vi "Plot Generator.vi"(7 "Frequency (Hz)":dbl, 8 "Count in":i32, 9 "Noise Level":dbl, 10 "Amplitude":dbl, 11 "DC":dbl) -> (2 "Numeric out":dbl)   [LabVIEW 2015]
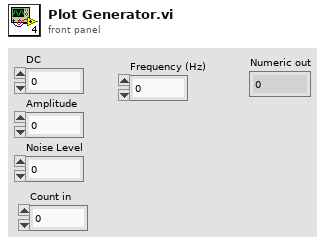
[diagram p1: front panel]
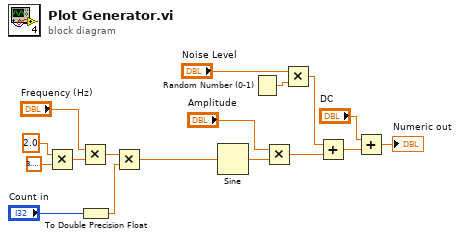
[diagram p0: block diagram]
diagram:
  n1 = Multiply(x=2.0, y=3.141592653589793) -> (x*y=w2:dbl)
  n2 = Multiply(x="Frequency (Hz)", y=w2) -> (x*y=w6:dbl)
  n3 = To Double Precision Float(number="Count in") -> (double precision float=w1:dbl)
  n4 = Multiply(x=w6, y=w1) -> (x*y=w7:dbl)
  n5 = Sine(x=w7) -> (sin(x)=w9:dbl)
  n6 = Random Number (0-1)() -> (number: 0 to 1=w12:dbl)
  n7 = Multiply(x="Amplitude", y=w9) -> (x*y=w10:dbl)
  n8 = Multiply(x="Noise Level", y=w12) -> (x*y=w13:dbl)
  n9 = Add(x=w13, y=w10) -> (x+y=w14:dbl)
  n10 = Add(x="DC", y=w14) -> (x+y=→"Numeric out":dbl)
